vi "Serial Port - Write Selected Names.vi"(8 "error in (no error)":errorcluster, 9 "Selected Names":string[](array[string]), 10 "COM Port List":string[](array[string]), 11 "Ctrl Refs in":refnum<vi>[](array[refnum])) -> (0 "error out":errorcluster, 3 "Selected Values":i32[](array[numeric]))   [LabVIEW 2011]
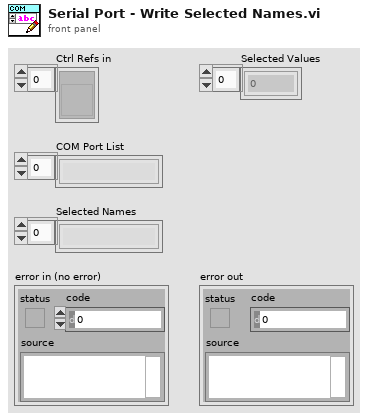
[diagram p1: front panel]
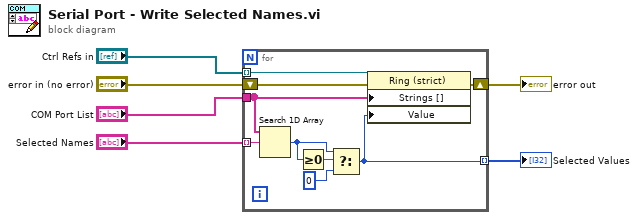
[diagram p0: block diagram]
diagram:
  n1 = for {
    tunnel: "COM Port List" -> [w11]
    tunnel: "Ctrl Refs in" -> [w15] mode=indexing
    shift-right: [w14] -> w2
    shift-left: "error in (no error)" -> [w13]
    tunnel: "Selected Names" -> [w12] mode=indexing
    tunnel: [w7] -> w1 mode=indexing
    n2 = Search 1D Array(1D array=w11, element=w12) -> (index of element=w9:i32)  [unwired: 1 in]
    n3 = Greater Or Equal To 0?(x=w9) -> (x >= 0?=w10:bool)
    n4 = Select(t=w9, s=w10, f=0) -> (s? t:f=w7:i32)
    n5 = property class="Ring (strict)"(reference=w15, error in=w13, "Strings []"=w11, "Value"=w7) -> (error out=w14:errorcluster)  [unwired: 1 out]
  }
  "error out" <- w2
  "Selected Values" <- w1
